vi "ProfilesTableControl.vi"(0 "CtlRef":refnum<vi>, 1 "Flow?":i32, 2 "Controller?":bool=TRUE, 5 "CharIn":i16, 7 "VKey":T1, 9 "ScanCode":i16) -> (4 "ColInsert?":bool, 6 "CharOut":i16, 15 "Discard?":bool)   [LabVIEW 2013]
uses:
  <vilib>/event_ctls.llb/eventvkey.ctl
  <vilib>/Utility/miscctls.llb/LVRowAndColumnTypeDef.ctl
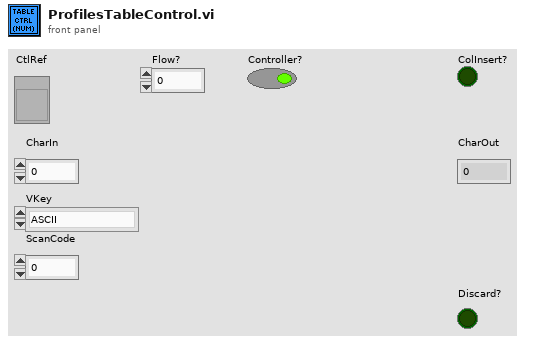
[diagram p1: front panel]
types:
  T1 = typedef "eventvkey.ctl" = enum16{"ASCII", "Enter", "Return", "Shift", "Ctrl", "Alt", "Cmd", "Opt", "Caps", "NumLock", "Clear", "Break", "Up", "Down", "Left", "Right", "Insert", "Delete", "Home", "End", "PageUp", "PageDown", "Escape", "Help", "Pause", "ScrollLock", "F1", "F2", "F3", "F4", "F5", "F6", "F7", "F8", "F9", "F10", "F11", "F12", "F13", "F14", "F15", "F16", "F17", "F18", "F19", "F20", "F21", "F22", "F23", "F24", "Play", "VolumeUp", "VolumeDown", "Mute", "Two Byte Char"}
  T2 = typedef "LVRowAndColumnTypeDef.ctl" = cluster{"Row":i32, "Column":i32}
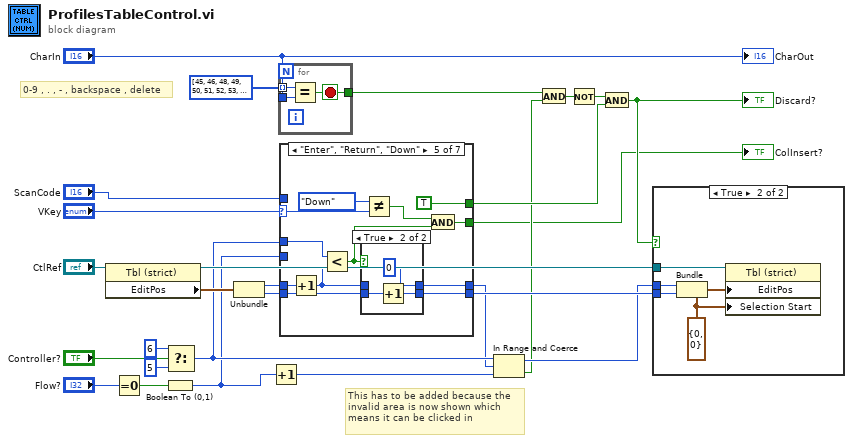
[diagram p0: block diagram]
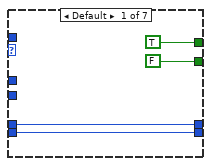
[diagram p3: hidden frame]
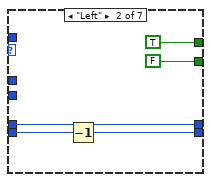
[diagram p4: hidden frame]
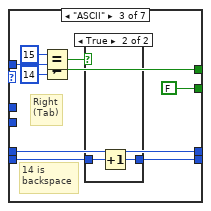
[diagram p5: hidden frame]
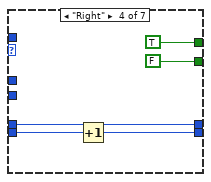
[diagram p7: hidden frame]
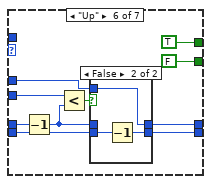
[diagram p9: hidden frame]
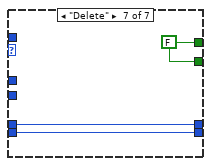
[diagram p11: hidden frame]
diagram:
  # "This has to be added because the\ninvalid area is now shown which\nmeans it can be clicked in"
  # "0-9 , . , - , backspace , delete"
  n1 = property on="Property Node" class="Tbl (strict)"(reference="CtlRef") -> (reference out=w24:refnum<vi>, "EditPos"=w23:T2)  [unwired: 1 in, 1 out]
  n2 = Equal To 0?(x="Flow?") -> (x = 0?=w4:bool)
  n3 = Boolean To (0,1)(Boolean=w4) -> (0, 1=w2:i16)
  n4 = Select(t=6, s="Controller?", f=5) -> (s? t:f=w12:i32)
  n5 = Unbundle(w23) -> ("Row"=w22:i32, "Column"=w21:i32)
  n6 = Increment(x=w2) -> (x+1=w9:i16)
  n7 = for {
    tunnel: i16[] [45, 46, 48, 49, 50, 51, 52, 53, 54, 55, 56, 57] -> [w30] mode=indexing
    tunnel: "CharIn" -> [w29]
    tunnel: [w28] -> w5
    stop <- w28 stop-if-true
    n8 = Equal?(x=w30, y=w29) -> (x = y?=w28:bool)
  }
  n9 = case shown="\"Enter\", \"Return\", \"Down\"" "VKey" {
    selector: "VKey" -> [_ _ _ _ w61 _ _]
    tunnel: "ScanCode" -> [_ _ w43 _ _ _ _]
    tunnel: w22 -> [w34 w37 w45 w54 w67 w83 w91]
    tunnel: w21 -> [w33 w39 w46 w56 w66 w77 w90]
    tunnel: [w34 w37 w45 w54 w65 w80 w91] -> w11
    tunnel: [w33 w38 w44 w55 w64 w79 w90] -> w20
    tunnel: w12 -> [_ _ _ _ w63 w75 _]
    tunnel: [TRUE TRUE w41 TRUE TRUE TRUE w89] -> w16
    tunnel: w2 -> [_ _ _ _ _ w76 _]
    tunnel: [FALSE FALSE FALSE FALSE w58 FALSE w89] -> w1
    frame Default {
    }
    frame "Left" {
      n10 = Decrement(x=w39) -> (x-1=w38:i32)
    }
    frame "ASCII" {
      # "14 is\nbackspace"
      # "Right\n(Tab)"
      n11 = Equal?(x=i16 15, y=w43) -> (x = y?=w47:bool)
      n12 = Not Equal?(x=w43, y=i16 14 ("x")) -> (x != y?=w41:bool)
      n13 = case shown="True" w47 {
        tunnel: w46 -> [w49 w51]
        tunnel: [w49 w50] -> w44
        frame False {
        }
        frame True {
          n14 = Increment(x=w51) -> (x+1=w50:i32)
        }
      }
    }
    frame "Right" {
      n15 = Increment(x=w56) -> (x+1=w55:i32)
    }
    frame "Enter", "Return", "Down" {
      n16 = Increment(x=w67) -> (x+1=w68:i32)
      n17 = Less?(x=w63, y=w68) -> (x < y?=w57:bool)
      n18 = case shown="True" w57 {
        tunnel: w68 -> [w70 _]
        tunnel: w66 -> [w69 w73]
        tunnel: [w70 0] -> w65
        tunnel: [w69 w72] -> w64
        frame False {
        }
        frame True {
          n19 = Increment(x=w73) -> (x+1=w72:i32)
        }
      }
      n20 = Not Equal?(x=eventvkey."Down", y=w61) -> (x != y?=w59:bool)
      n21 = And(x=w59, y=w57) -> (x .and. y?=w58:bool)
    }
    frame "Up" {
      n22 = Decrement(x=w83) -> (x-1=w78:i32)
      n23 = Less?(x=w76, y=w78) -> (x < y?=w81:bool)
      n24 = case shown="False" w81 {
        tunnel: w78 -> [w85 _]
        tunnel: w77 -> [w84 w88]
        tunnel: [w85 w86] -> w80
        tunnel: [w84 w87] -> w79
        tunnel: w75 -> [_ w86]
        frame True {
        }
        frame False {
          n25 = Decrement(x=w88) -> (x-1=w87:i32)
        }
      }
    }
    frame "Delete" {
      w89 = FALSE
    }
  }
  "ColInsert?" <- w1
  n26 = In Range and Coerce(upper limit=w12, x=w11, lower limit=w9) -> (coerced(x)=w10:i32, In Range?=w6:bool)
  n27 = And(x=w5, y=w6) -> (x .and. y?=w8:bool)
  n28 = Not(x=w8) -> (.not. x?=w7:bool)
  n29 = And(x=w7, y=w16) -> (x .and. y?=w17:bool)
  "Discard?" <- w17
  n30 = case shown="True" w17 {
    tunnel: w24 -> [_ w96]
    tunnel: w10 -> [_ w94]
    tunnel: w20 -> [_ w93]
    frame False {
    }
    frame True {
      w92 = T2 {"Row"=0, "Column"=0} ("Active Cell:Active Cell")
      n31 = Bundle(cluster=w92, "Row"=w94, "Column"=w93) -> (w95:T2)
      n32 = property on="Property Node" class="Tbl (strict)"(reference=w96, "EditPos"=w95, "Selection Start"=w92) -> ()  [unwired: 1 in, 2 out]
    }
  }
  "CharOut" <- "CharIn"
